vi "Brake Test Project.vi"() -> ()   [LabVIEW 2017]
uses:
  <vilib>/Utility/file.llb/Read Delimited Spreadsheet (DBL).vi
  <vilib>/Utility/file.llb/Read Delimited Spreadsheet (string).vi
panel:
  out "o/p vs (I,%ef,T,N)":cluster{dbl[], "all rows":dbl[]}[](graph)
  out "Torquw vs Speed":cluster{dbl[], "all rows":dbl[]}(graph)
  out "o/p vs Speed":cluster{dbl[], "all rows":dbl[]}(graph)
  out "o/p vs Torque":cluster{dbl[], "all rows":dbl[]}(graph)
  out "o/p vs %efficiency":cluster{dbl[], "all rows":dbl[]}(graph)
  out "o/p vs Ioad current":cluster{dbl[], "all rows":dbl[]}(graph)
  out "N":dbl[](array[numeric])
  out "R(m)":dbl[](array[numeric])
  out "W2":dbl[](array[numeric])
  out "W1":dbl[](array[numeric])
  out "Current":dbl[](array[numeric])
  out "Voltage":dbl[](array[numeric])
  in  "?":bool
  out "Torque":dbl[](array[numeric])
  out "Input Power":dbl[](array[numeric])
  out "Output Power":dbl[](array[numeric])
  out "% Efficiency":dbl[](array[numeric])
  out "Input values":dbl[][](array[numeric])
  out "first row":string[](array[string])
  in  "file path (dialog if empty)":path
  # "BRAKE TEST"
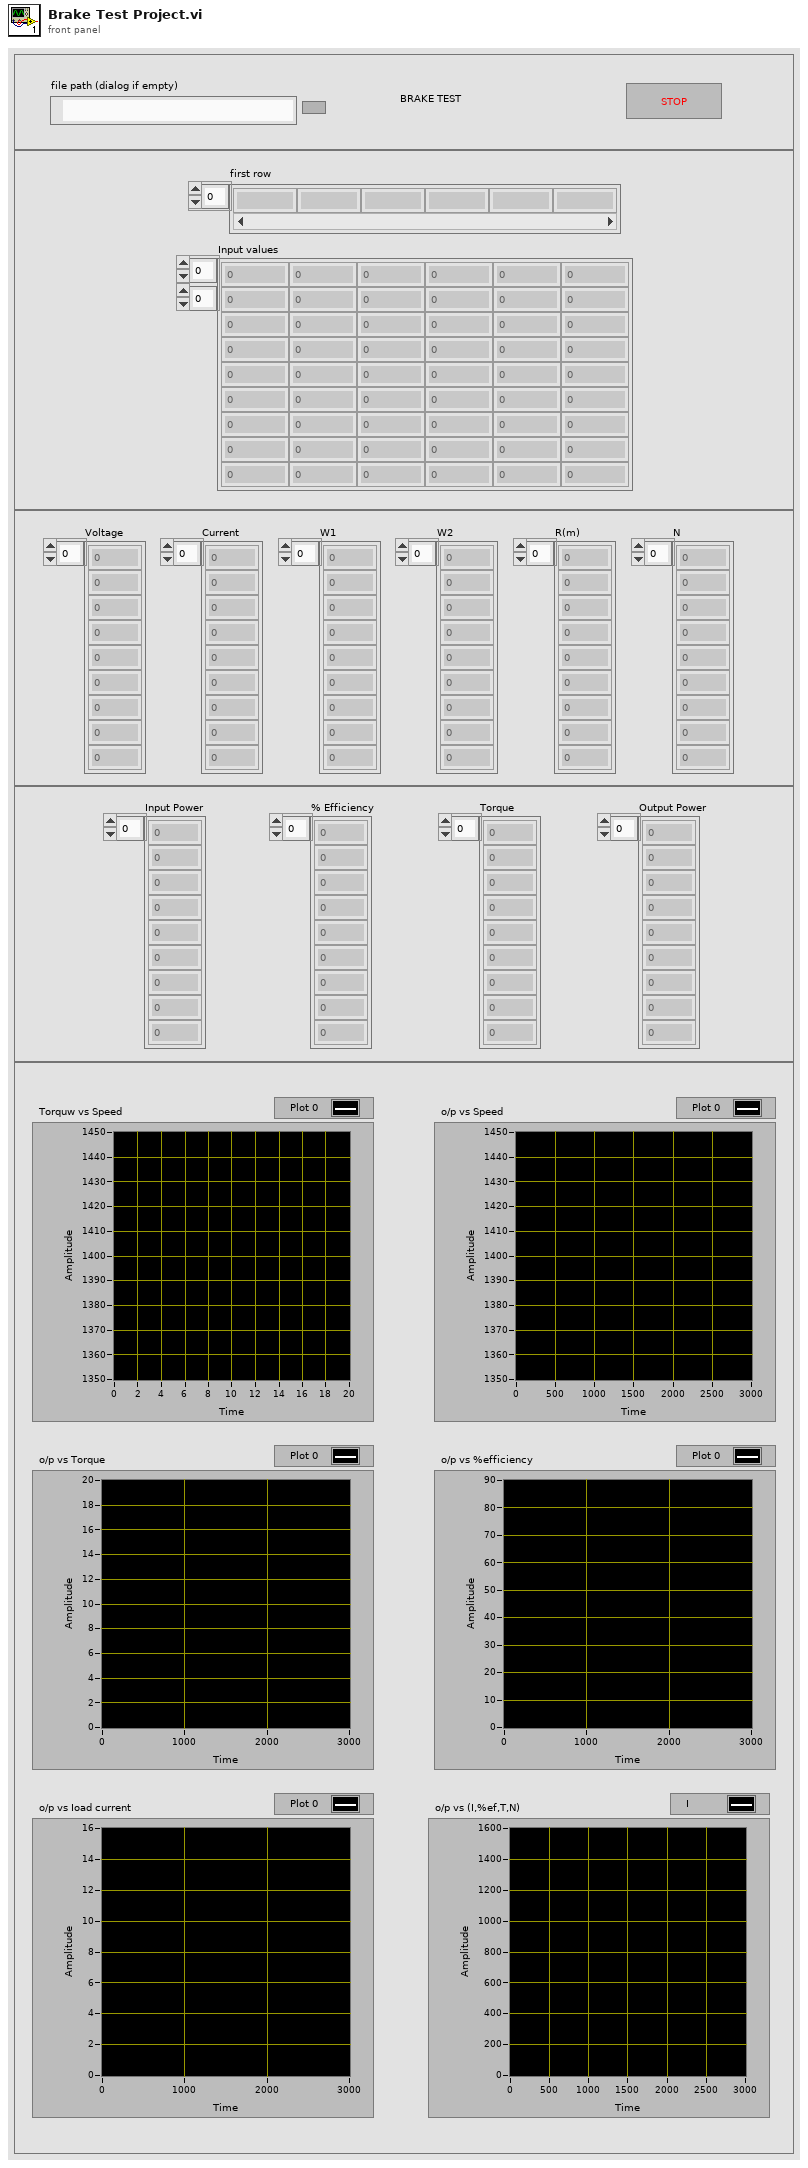
[diagram p1: front panel]
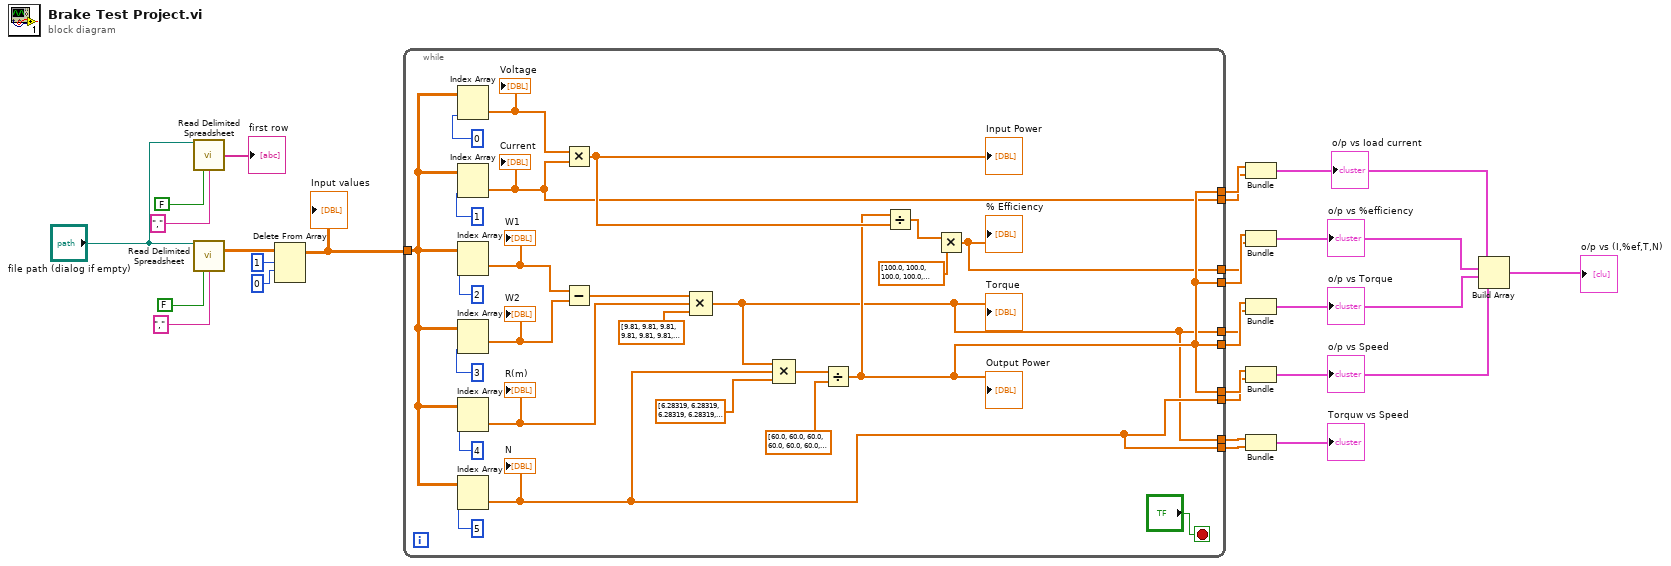
[diagram p0: block diagram]
diagram:
  n1 = call-poly <vilib>:"Read Delimited Spreadsheet.vi"("file path (dialog if empty)"="file path (dialog if empty)", "transpose? (F)"=FALSE, "delimiter (\\t)"="," ("delimiter (\\t)")) -> ("first row"=→"first row":string[])  [unwired: 7 in, 5 out]
  n2 = call-poly <vilib>:"Read Delimited Spreadsheet.vi"("file path (dialog if empty)"="file path (dialog if empty)", "transpose? (F)"=FALSE, "delimiter (\\t)"="," ("delimiter (\\t)")) -> ("all rows"=w20:dbl[][])  [unwired: 7 in, 5 out]
  n3 = Delete From Array(array=w20, length=1 ("index (row)"), index (row)=0 ("disabled index (col)")) -> (array with subset deleted=w17:dbl[][])  [unwired: 1 in, 1 out]
  "Input values" <- w17
  n4 = while {
    tunnel: w17 -> [w44]
    tunnel: [w31] -> w16
    tunnel: [w29] -> w15
    tunnel: [w31] -> w14
    tunnel: [w32] -> w13
    tunnel: [w31] -> w12
    tunnel: [w28] -> w11
    tunnel: [w31] -> w10
    tunnel: [w30] -> w9
    tunnel: [w29] -> w8
    tunnel: [w32] -> w7
    stop <- "?" stop-if-true
    n5 = Index Array(array=w44, index (col)=0 ("disabled index (col)")) -> (element=w43:dbl[])  [unwired: 1 in]
    "Voltage" <- w43
    n6 = Index Array(array=w44, index (col)=1 ("disabled index (col)")) -> (element=w30:dbl[])  [unwired: 1 in]
    "Current" <- w30
    n7 = Index Array(array=w44, index (col)=2 ("disabled index (col)")) -> (element=w41:dbl[])  [unwired: 1 in]
    "W1" <- w41
    n8 = Index Array(array=w44, index (col)=3 ("disabled index (col)")) -> (element=w42:dbl[])  [unwired: 1 in]
    "W2" <- w42
    n9 = Index Array(array=w44, index (col)=4 ("disabled index (col)")) -> (element=w34:dbl[])  [unwired: 1 in]
    "R(m)" <- w34
    n10 = Index Array(array=w44, index (col)=5 ("disabled index (col)")) -> (element=w32:dbl[])  [unwired: 1 in]
    "N" <- w32
    n11 = Multiply(x=w43, y=w30) -> (x*y=w33:dbl[])
    "Input Power" <- w33
    n12 = Subtract(x=w41, y=w42) -> (x-y=w40:dbl[])
    n13 = Compound Arithmetic op=MULTIPLY(w40, w34, dbl[] [9.81, 9.81, 9.81, 9.81, 9.81, 9.81, 9.81, 9.81, 9.81] ("value")) -> (w29:dbl[])
    "Torque" <- w29
    n14 = Compound Arithmetic op=MULTIPLY(w29, w32, dbl[] [6.28319, 6.28319, 6.28319, 6.28319, 6.28319, 6.28319, 6.28319, 6.28319, 6.28319] ("value")) -> (w37:dbl[])
    n15 = Divide(x=w37, y=dbl[] [60.0, 60.0, 60.0, 60.0, 60.0, 60.0, 60.0, 60.0, 60.0] ("value")) -> (x/y=w31:dbl[])
    "Output Power" <- w31
    n16 = Divide(x=w31, y=w33) -> (x/y=w35:dbl[])
    n17 = Multiply(x=w35, y=dbl[] [100.0, 100.0, 100.0, 100.0, 100.0, 100.0, 100.0, 100.0, 100.0] ("value")) -> (x*y=w28:dbl[])
    "% Efficiency" <- w28
  }
  n18 = Bundle(w10, "all rows"=w9) -> (w5:cluster{dbl[], "all rows":dbl[]})  [unwired: 1 in]
  "o/p vs Ioad current" <- w5
  n19 = Bundle(w12, w11) -> (w4:cluster{dbl[], dbl[]})  [unwired: 1 in]
  "o/p vs %efficiency" <- w4
  n20 = Bundle(w16, w15) -> (w3:cluster{dbl[], dbl[]})  [unwired: 1 in]
  "o/p vs Torque" <- w3
  n21 = Bundle(w14, "all rows"=w13) -> (w2:cluster{dbl[], "all rows":dbl[]})  [unwired: 1 in]
  "o/p vs Speed" <- w2
  n22 = Bundle(w8, "all rows"=w7) -> (→"Torquw vs Speed":cluster{dbl[], "all rows":dbl[]})  [unwired: 1 in]
  n23 = Build Array(w5, w4, w3, w2) -> (→"o/p vs (I,%ef,T,N)":cluster{dbl[], "all rows":dbl[]}[])
